vi "Single.vi"() -> ()   [LabVIEW 2017]
doc: "SubVI criada para testar o funcionamento do caso Single Player"
uses:
  controls/DataOut.ctl
  controls/Tabuleiro.ctl
  controls/GameOption.ctl
  controls/States.ctl
  controls/DataIn.ctl
  controls/LogStates.ctl
  controls/TabuleiroCoordenadas.ctl
panel:
  in  "Reiniciar":bool
  in  "Sair":bool
  out "Quem joga":string
  out "Tabuleiro":T1
  out "DataOut":T2
  # "JOGO DA VELHA"
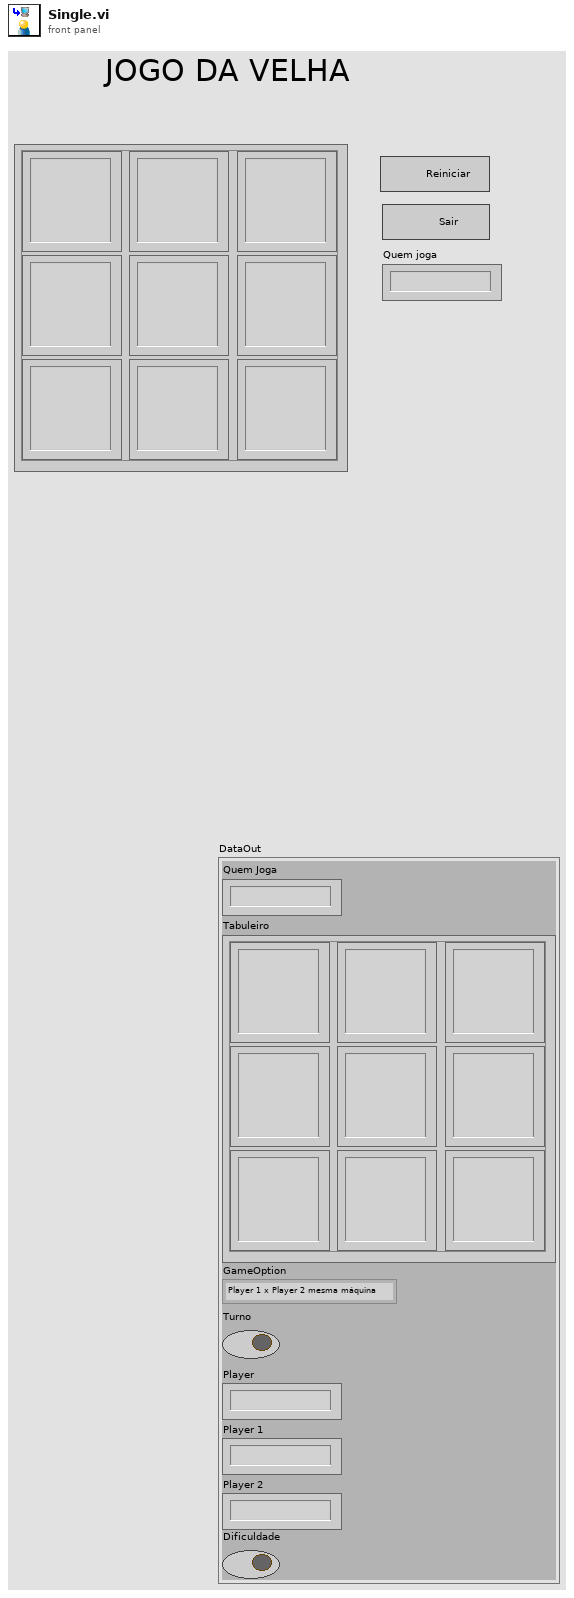
[diagram p1: front panel]
types:
  T1 = typedef "Tabuleiro.ctl" = cluster{"(0,0)":string, "(1,0)":string, "(0,1)":string, "(1,1)":string, "(2,0)":string, "(1,2)":string, "(2,2)":string, "(0,2)":string, "(2,1) ":string}
  T2 = typedef "DataOut.ctl" = cluster{"Quem Joga":string, "Tabuleiro":T1, "GameOption":T3, "Turno":bool, "Player":string, "Player 1":string, "Player 2":string, "Dificuldade":bool}
  T3 = typedef "GameOption.ctl" = enum16{"Player 1 x Player 2 mesma máquina", "Player 1 x Player 2 pela rede", "Player 1 x Computador", "Wait for Event", "Initialize"}
  T4 = typedef "States.ctl" = enum16{"Initialize", "Player (wait for event)", "Stop", "PC", "Restart"}
  T5 = typedef "DataIn.ctl" = cluster{"Quem Joga":string, "Tabuleiro":T1, "GameOption":T3, "Turno":bool, "Player":string, "Player 1":string, "Player 2":string, "Dificuldade":bool}
  T6 = typedef "LogStates.ctl" = enum16{"Initialize", "Write", "Write (win, draw)", "Write (PC first)", "Write (Player first)", "Close"}
  T7 = typedef "TabuleiroCoordenadas.ctl" = enum16{"0,0", "0,1", "0,2", "1,0", "1,1", "1,2", "2,0", "2,1", "2,2"}
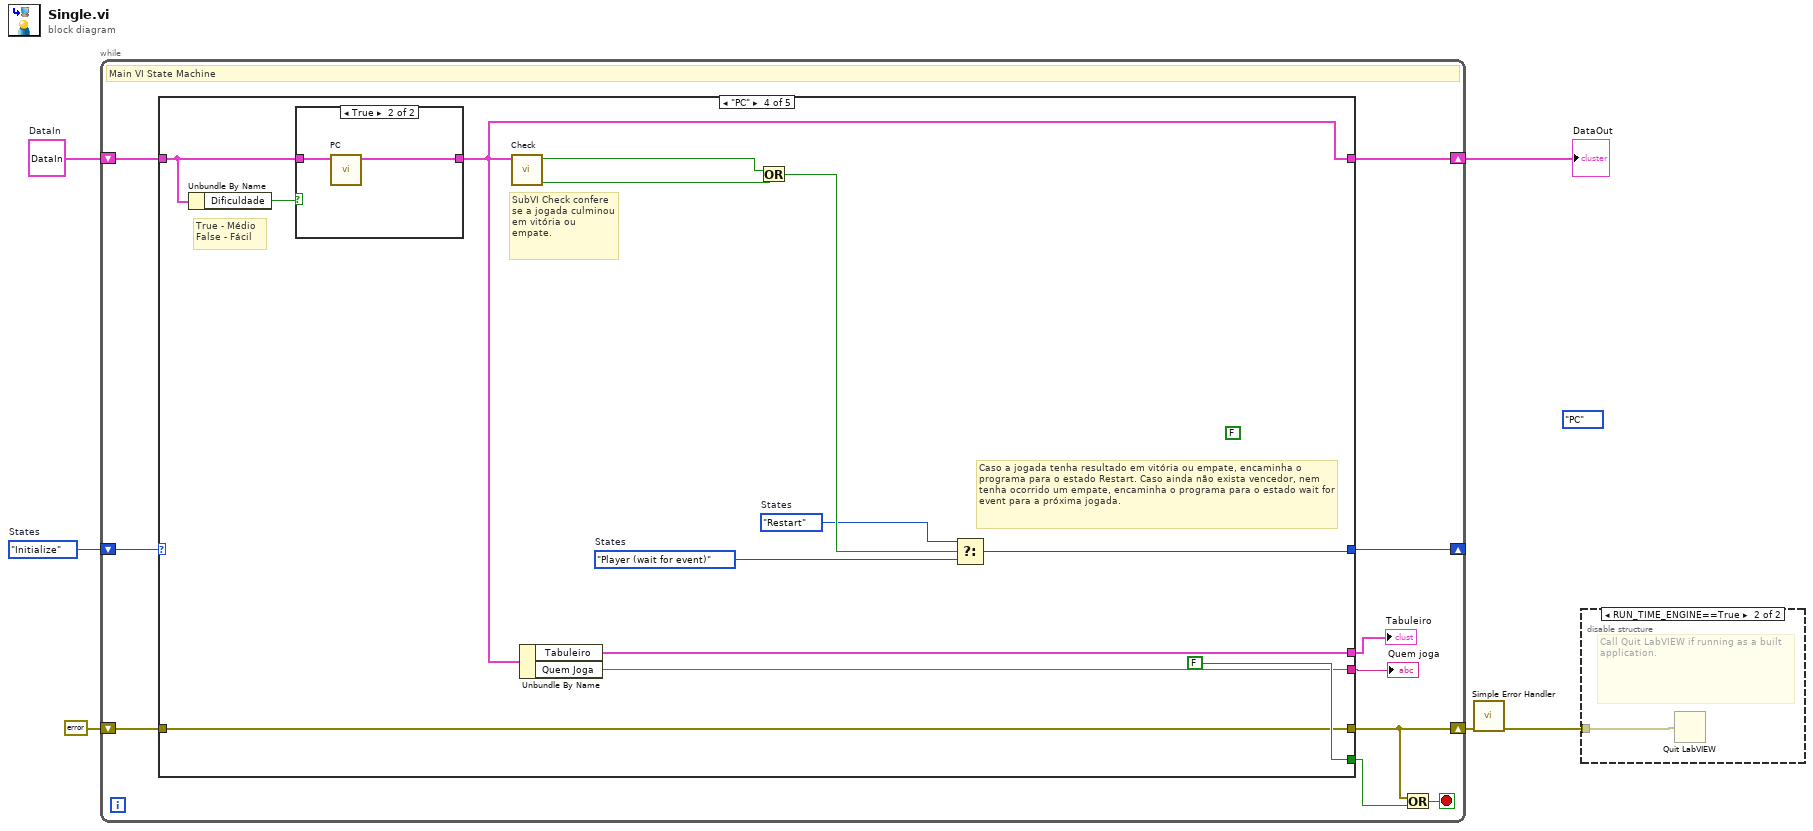
[diagram p0: block diagram]
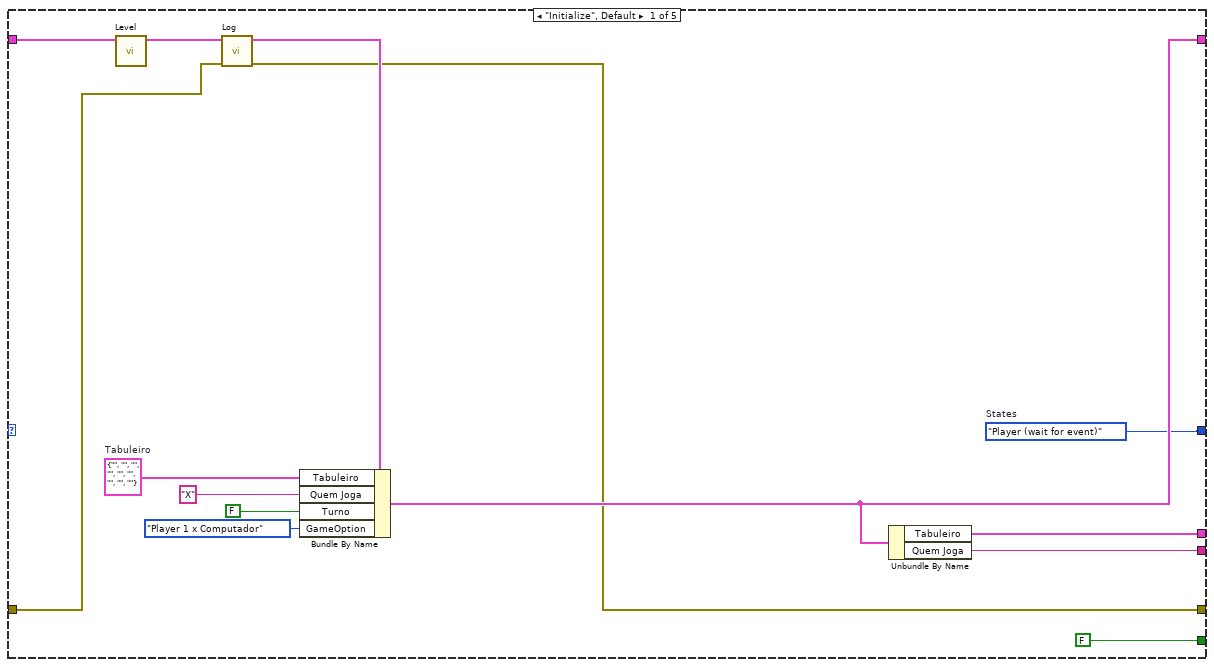
[diagram p3: hidden frame]
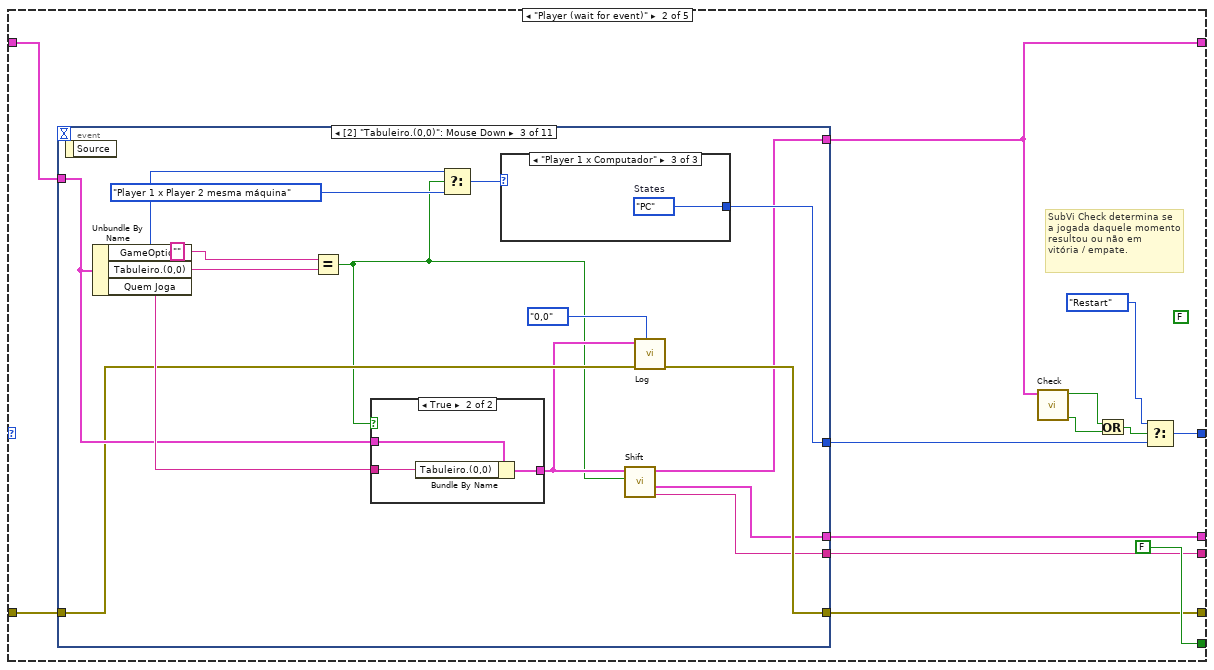
[diagram p4: hidden frame]
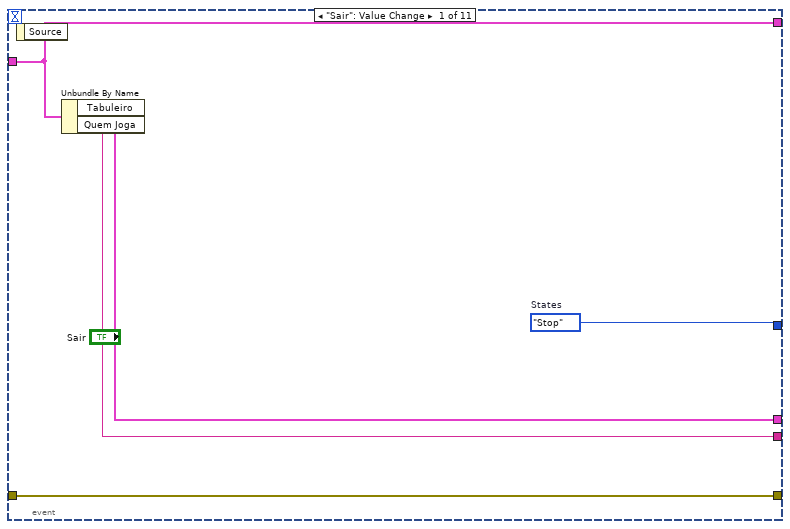
[diagram p5: hidden frame]
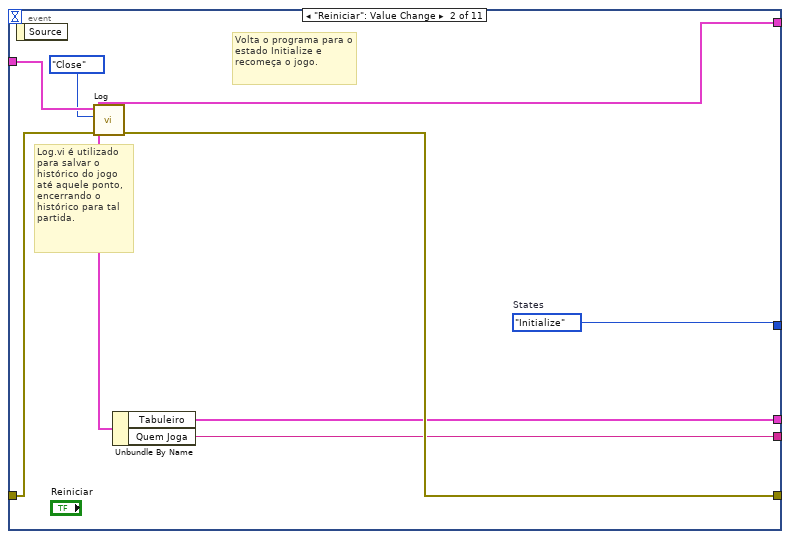
[diagram p6: hidden frame]
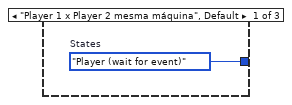
[diagram p8: hidden frame]
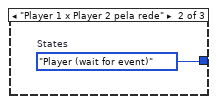
[diagram p9: hidden frame]
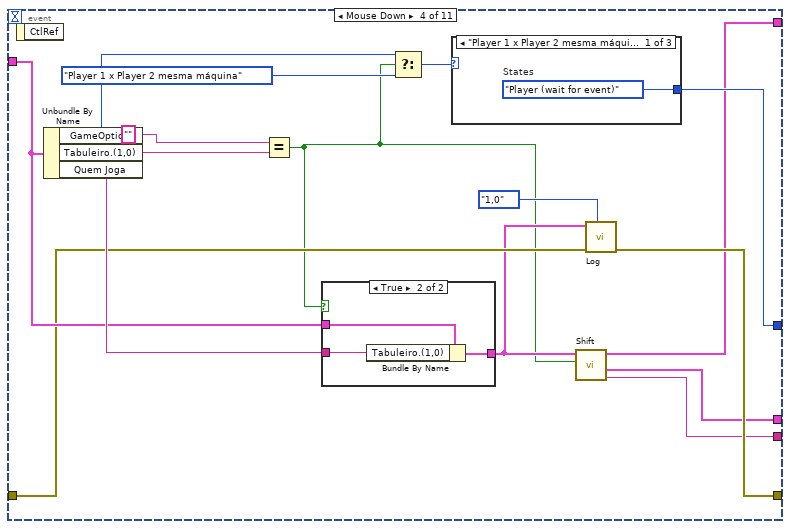
[diagram p10: hidden frame]
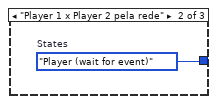
[diagram p12: hidden frame]
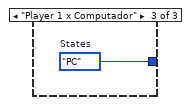
[diagram p13: hidden frame]
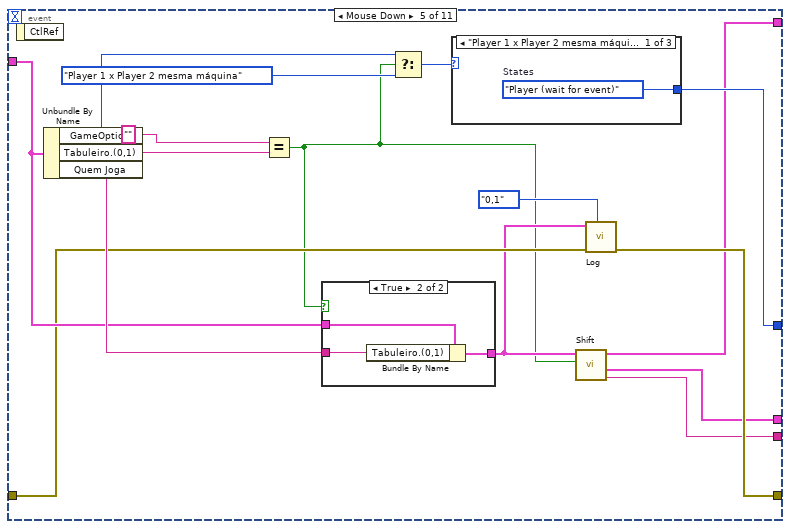
[diagram p14: hidden frame]
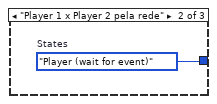
[diagram p16: hidden frame]
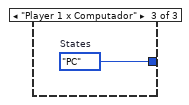
[diagram p17: hidden frame]
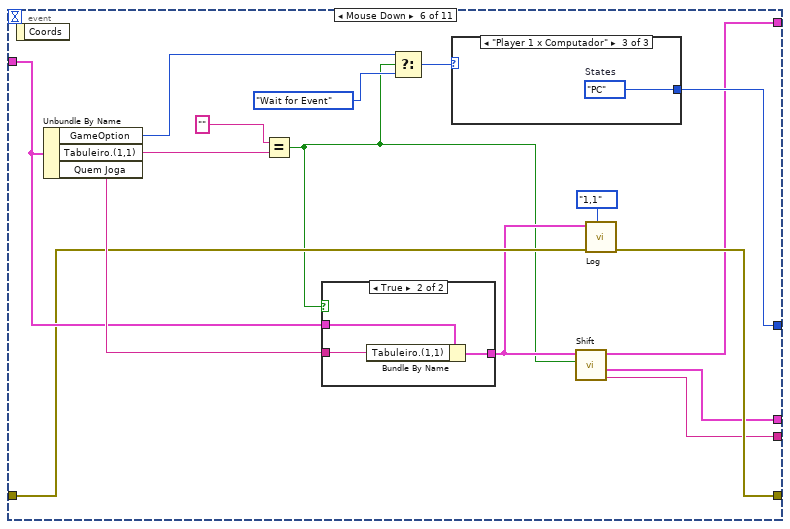
[diagram p18: hidden frame]
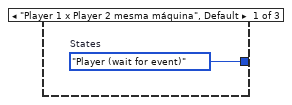
[diagram p20: hidden frame]
diagram:
  (unwired) States."PC" ("f")
  w4 = T5 {"Quem Joga"="", "Tabuleiro"={"(0,0)"="", "(1,0)"="", "(0,1)"="", "(1,1)"="", "(2,0)"="", "(1,2)"="", "(2,2)"="", "(0,2)"="", "(2,1) "=""}, "GameOption"=enum."Player 1 x Player 2 mesma máquina", "Turno"=FALSE, "Player"="", "Player 1"="", "Player 2"="", "Dificuldade"=FALSE}  # DataIn
  w5 = States."Initialize"  # States
  n1 = while {
    shift-right: [w13] -> w6
    shift-left: w4 -> [w14]
    shift-right: [w11] -> w3
    shift-left: errorcluster {"status"=FALSE, "code"=0, "source"=""} ("error constant") -> [w12]
    shift-right: [w10] -> _
    shift-left: w5 -> [w15]
    stop <- w16 stop-if-true
    # "Main VI State Machine"
    n2 = case shown="\"PC\"" w15 {
      tunnel: w14 -> [w18 w42 w267 w271 w296]
      tunnel: [w27 w31 w267 w272 w287] -> w13
      tunnel: w12 -> [w20 w41 w269 w273 w295]
      tunnel: [w19 w40 w269 w273 w288] -> w11
      tunnel: [w23 w36 w268 w276 w289] -> w10
      tunnel: [w26 w39 w266 w275 w293] -> w9
      tunnel: [w25 w38 w265 w274 w292] -> w8
      tunnel: [FALSE FALSE TRUE FALSE FALSE] -> w7
      frame "Initialize", Default {
        w23 = States."Player (wait for event)"  # States
        w28 = T1 {"(0,0)"="", "(1,0)"="", "(0,1)"="", "(1,1)"="", "(2,0)"="", "(1,2)"="", "(2,2)"="", "(0,2)"="", "(2,1) "=""}  # Tabuleiro
        n3 = call "Level.vi"("DataIn"=w18) -> ("Cluster"=w17:T2)  [unwired: 10 in]
        n4 = call "Log.vi"("Error In"=w20, "DataIn"=w17) -> ("Error Out"=w19:errorcluster, "DataOut"=w21:T2)  [unwired: 8 in]
        n5 = Bundle By Name(cluster=w21, "Tabuleiro"=w28, "Quem Joga"="X", "Turno"=FALSE, "GameOption"=GameOption."Player 1 x Computador") -> (w27:T2)
        n6 = Unbundle By Name(w27) -> ("Tabuleiro"=w25:T1, "Quem Joga"=w26:string)
      }
      frame "Player (wait for event)" {
        (unwired) FALSE ("Nível")
        # "SubVi Check determina se a jogada daquele momento resultou ou não em vitória / empate."
        n7 = event shown="[2] \"Tabuleiro.(0,0)\": Mouse Down" {
          selector: _ -> [_ _ _ _ _ _ _ _ _ _ _]
          dyn-events: _ -> [_ _ _ _ _ _ _ _ _ _ _]
          timeout: _ -> [_ _ _ _ _ _ _ _ _ _ _]
          tunnel: w42 -> [w48 w55 w65 w88 w111 w135 w157 w180 w203 w226 w249]
          tunnel: [w48 w51 w60 w83 w106 w130 w152 w175 w198 w221 w244] -> w31
          tunnel: w41 -> [w47 w53 w63 w86 w109 w133 w155 w178 w201 w224 w247]
          tunnel: [w47 w52 w62 w85 w108 w132 w154 w177 w200 w223 w246] -> w40
          tunnel: [w46 w50 w59 w82 w105 w129 w151 w174 w197 w220 w243] -> w38
          tunnel: [w45 w49 w58 w81 w104 w128 w150 w173 w196 w219 w242] -> w39
          tunnel: [w44 w56 w67 w90 w113 w137 w159 w182 w205 w228 w251] -> w37
          event "Sair": Value Change {
            w44 = States."Stop"  # States
            n8 = event-data() -> ()  [unwired: 1 in, 1 out]
            n9 = Unbundle By Name(w48) -> ("Tabuleiro"=w46:T1, "Quem Joga"=w45:string)
          }
          event "Reiniciar": Value Change {
            w56 = States."Initialize"  # States
            # "Log.vi é utilizado para salvar o histórico do jogo até aquele ponto, encerrando o histórico para tal partida."
            # "Volta o programa para o estado Initialize e recomeça o jogo."
            n10 = event-data() -> ()  [unwired: 1 in, 1 out]
            n11 = call "Log.vi"("Error In"=w53, "Log States"=LogStates."Close", "DataIn"=w55) -> ("Error Out"=w52:errorcluster, "DataOut"=w51:T2)  [unwired: 7 in]
            n12 = Unbundle By Name(w51) -> ("Tabuleiro"=w50:T1, "Quem Joga"=w49:string)
          }
          event Mouse Down {
            n13 = event-data() -> ()  [unwired: 1 in, 1 out]
            n14 = Unbundle By Name(w65) -> ("GameOption"=w69:T3, "Tabuleiro.(0,0)"=w72:string, "Quem Joga"=w66:string)
            n15 = Equal?(x="", y=w72) -> (x = y?=w57:bool)
            n16 = case shown="True" w57 {
              tunnel: w66 -> [_ w75]
              tunnel: w65 -> [w73 w76]
              tunnel: [w73 w74] -> w61
              frame False {
              }
              frame True {
                n17 = Bundle By Name(cluster=w76, "Tabuleiro.(0,0)"=w75) -> (w74:T2)
              }
            }
            n18 = Select(t=w69, s=w57, f=GameOption."Player 1 x Player 2 mesma máquina") -> (s? t:f=w68:T3)
            n19 = case shown="\"Player 1 x Computador\"" w68 {
              tunnel: [w77 w78 w79] -> w67
              frame "Player 1 x Player 2 mesma máquina", Default {
                w77 = States."Player (wait for event)"  # States
              }
              frame "Player 1 x Player 2 pela rede" {
                w78 = States."Player (wait for event)"  # States
              }
              frame "Player 1 x Computador" {
                w79 = States."PC"  # States
              }
            }
            n20 = call "Shift.vi"("Confirmação"=w57, "DataIn"=w61) -> ("Turno"=w58:string, "Tabuleiro"=w59:T1, "DataOut"=w60:T2)  [unwired: 7 in]
            n21 = call "Log.vi"("Enum Coordenadas"=TabuleiroCoordenadas."0,0" ("Enum"), "Error In"=w63, "DataIn"=w61) -> ("Error Out"=w62:errorcluster)  [unwired: 7 in, 1 out]
          }
          event Mouse Down {
            n22 = event-data() -> ()  [unwired: 1 in, 1 out]
            n23 = Unbundle By Name(w88) -> ("GameOption"=w92:T3, "Tabuleiro.(1,0)"=w95:string, "Quem Joga"=w89:string)
            n24 = Equal?(x="", y=w95) -> (x = y?=w80:bool)
            n25 = case shown="True" w80 {
              tunnel: w89 -> [_ w98]
              tunnel: w88 -> [w96 w99]
              tunnel: [w96 w97] -> w84
              frame False {
              }
              frame True {
                n26 = Bundle By Name(cluster=w99, "Tabuleiro.(1,0)"=w98) -> (w97:T2)
              }
            }
            n27 = Select(t=w92, s=w80, f=GameOption."Player 1 x Player 2 mesma máquina") -> (s? t:f=w91:T3)
            n28 = case shown="\"Player 1 x Player 2 mesma máquina\", Default" w91 {
              tunnel: [w100 w101 w102] -> w90
              frame "Player 1 x Player 2 mesma máquina", Default {
                w100 = States."Player (wait for event)"  # States
              }
              frame "Player 1 x Player 2 pela rede" {
                w101 = States."Player (wait for event)"  # States
              }
              frame "Player 1 x Computador" {
                w102 = States."PC"  # States
              }
            }
            n29 = call "Shift.vi"("Confirmação"=w80, "DataIn"=w84) -> ("Turno"=w81:string, "Tabuleiro"=w82:T1, "DataOut"=w83:T2)  [unwired: 7 in]
            n30 = call "Log.vi"("Enum Coordenadas"=TabuleiroCoordenadas."1,0" ("Enum"), "Error In"=w86, "DataIn"=w84) -> ("Error Out"=w85:errorcluster)  [unwired: 7 in, 1 out]
          }
          event Mouse Down {
            n31 = event-data() -> ()  [unwired: 1 in, 1 out]
            n32 = Unbundle By Name(w111) -> ("GameOption"=w115:T3, "Tabuleiro.(0,1)"=w118:string, "Quem Joga"=w112:string)
            n33 = Equal?(x="", y=w118) -> (x = y?=w103:bool)
            n34 = case shown="True" w103 {
              tunnel: w112 -> [_ w121]
              tunnel: w111 -> [w119 w122]
              tunnel: [w119 w120] -> w107
              frame False {
              }
              frame True {
                n35 = Bundle By Name(cluster=w122, "Tabuleiro.(0,1)"=w121) -> (w120:T2)
              }
            }
            n36 = Select(t=w115, s=w103, f=GameOption."Player 1 x Player 2 mesma máquina") -> (s? t:f=w114:T3)
            n37 = case shown="\"Player 1 x Player 2 mesma máquina\", Default" w114 {
              tunnel: [w123 w124 w125] -> w113
              frame "Player 1 x Player 2 mesma máquina", Default {
                w123 = States."Player (wait for event)"  # States
              }
              frame "Player 1 x Player 2 pela rede" {
                w124 = States."Player (wait for event)"  # States
              }
              frame "Player 1 x Computador" {
                w125 = States."PC"  # States
              }
            }
            n38 = call "Shift.vi"("Confirmação"=w103, "DataIn"=w107) -> ("Turno"=w104:string, "Tabuleiro"=w105:T1, "DataOut"=w106:T2)  [unwired: 7 in]
            n39 = call "Log.vi"("Enum Coordenadas"=TabuleiroCoordenadas."0,1" ("Enum"), "Error In"=w109, "DataIn"=w107) -> ("Error Out"=w108:errorcluster)  [unwired: 7 in, 1 out]
          }
          event Mouse Down {
            n40 = event-data() -> ()  [unwired: 1 in, 1 out]
            n41 = Unbundle By Name(w135) -> ("GameOption"=w126:T3, "Tabuleiro.(1,1)"=w141:string, "Quem Joga"=w136:string)
            n42 = Equal?(x="", y=w141) -> (x = y?=w127:bool)
            n43 = case shown="True" w127 {
              tunnel: w136 -> [_ w144]
              tunnel: w135 -> [w142 w145]
              tunnel: [w142 w143] -> w131
              frame False {
              }
              frame True {
                n44 = Bundle By Name(cluster=w145, "Tabuleiro.(1,1)"=w144) -> (w143:T2)
              }
            }
            n45 = Select(t=w126, s=w127, f=GameOption."Wait for Event") -> (s? t:f=w138:T3)
            n46 = case shown="\"Player 1 x Computador\"" w138 {
              tunnel: [w146 w147 w148] -> w137
              frame "Player 1 x Player 2 mesma máquina", Default {
                w146 = States."Player (wait for event)"  # States
              }
              frame "Player 1 x Player 2 pela rede" {
                w147 = States."Player (wait for event)"  # States
              }
              frame "Player 1 x Computador" {
                w148 = States."PC"  # States
              }
            }
            n47 = call "Shift.vi"("Confirmação"=w127, "DataIn"=w131) -> ("Turno"=w128:string, "Tabuleiro"=w129:T1, "DataOut"=w130:T2)  [unwired: 7 in]
            n48 = call "Log.vi"("Enum Coordenadas"=TabuleiroCoordenadas."1,1" ("Enum"), "Error In"=w133, "DataIn"=w131) -> ("Error Out"=w132:errorcluster)  [unwired: 7 in, 1 out]
          }
          event Mouse Down {
            n49 = event-data() -> ()  [unwired: 1 in, 1 out]
            n50 = Unbundle By Name(w157) -> ("GameOption"=w161:T3, "Tabuleiro.(2,0)"=w164:string, "Quem Joga"=w158:string)
            n51 = Equal?(x="", y=w164) -> (x = y?=w149:bool)
            n52 = case shown="True" w149 {
              tunnel: w158 -> [_ w167]
              tunnel: w157 -> [w165 w168]
              tunnel: [w165 w166] -> w153
              frame False {
              }
              frame True {
                n53 = Bundle By Name(cluster=w168, "Tabuleiro.(2,0)"=w167) -> (w166:T2)
              }
            }
            n54 = Select(t=w161, s=w149, f=GameOption."Player 1 x Player 2 mesma máquina") -> (s? t:f=w160:T3)
            n55 = case shown="\"Player 1 x Player 2 mesma máquina\", Default" w160 {
              tunnel: [w169 w170 w171] -> w159
              frame "Player 1 x Player 2 mesma máquina", Default {
                w169 = States."Player (wait for event)"  # States
              }
              frame "Player 1 x Player 2 pela rede" {
                w170 = States."Player (wait for event)"  # States
              }
              frame "Player 1 x Computador" {
                w171 = States."PC"  # States
              }
            }
            n56 = call "Shift.vi"("Confirmação"=w149, "DataIn"=w153) -> ("Turno"=w150:string, "Tabuleiro"=w151:T1, "DataOut"=w152:T2)  [unwired: 7 in]
            n57 = call "Log.vi"("Enum Coordenadas"=TabuleiroCoordenadas."2,0" ("Enum"), "Error In"=w155, "DataIn"=w153) -> ("Error Out"=w154:errorcluster)  [unwired: 7 in, 1 out]
          }
          event Mouse Down {
            n58 = event-data() -> ()  [unwired: 1 in, 1 out]
            n59 = Unbundle By Name(w180) -> ("GameOption"=w184:T3, "Tabuleiro.(1,2)"=w187:string, "Quem Joga"=w181:string)
            n60 = Equal?(x="", y=w187) -> (x = y?=w172:bool)
            n61 = case shown="True" w172 {
              tunnel: w181 -> [_ w190]
              tunnel: w180 -> [w188 w191]
              tunnel: [w188 w189] -> w176
              frame False {
              }
              frame True {
                n62 = Bundle By Name(cluster=w191, "Tabuleiro.(1,2)"=w190) -> (w189:T2)
              }
            }
            n63 = Select(t=w184, s=w172, f=GameOption."Player 1 x Player 2 mesma máquina") -> (s? t:f=w183:T3)
            n64 = case shown="\"Player 1 x Player 2 mesma máquina\", Default" w183 {
              tunnel: [w192 w193 w194] -> w182
              frame "Player 1 x Player 2 mesma máquina", Default {
                w192 = States."Player (wait for event)"  # States
              }
              frame "Player 1 x Player 2 pela rede" {
                w193 = States."Player (wait for event)"  # States
              }
              frame "Player 1 x Computador" {
                w194 = States."PC"  # States
              }
            }
            n65 = call "Shift.vi"("Confirmação"=w172, "DataIn"=w176) -> ("Turno"=w173:string, "Tabuleiro"=w174:T1, "DataOut"=w175:T2)  [unwired: 7 in]
            n66 = call "Log.vi"("Enum Coordenadas"=TabuleiroCoordenadas."1,2" ("Enum"), "Error In"=w178, "DataIn"=w176) -> ("Error Out"=w177:errorcluster)  [unwired: 7 in, 1 out]
          }
          event Mouse Down {
            n67 = event-data() -> ()  [unwired: 1 in, 1 out]
            n68 = Unbundle By Name(w203) -> ("GameOption"=w207:T3, "Tabuleiro.(2,2)"=w210:string, "Quem Joga"=w204:string)
            n69 = Equal?(x="", y=w210) -> (x = y?=w195:bool)
            n70 = case shown="True" w195 {
              tunnel: w204 -> [_ w213]
              tunnel: w203 -> [w211 w214]
              tunnel: [w211 w212] -> w199
              frame False {
              }
              frame True {
                n71 = Bundle By Name(cluster=w214, "Tabuleiro.(2,2)"=w213) -> (w212:T2)
              }
            }
            n72 = Select(t=w207, s=w195, f=GameOption."Player 1 x Player 2 mesma máquina") -> (s? t:f=w206:T3)
            n73 = case shown="\"Player 1 x Player 2 mesma máquina\", Default" w206 {
              tunnel: [w215 w216 w217] -> w205
              frame "Player 1 x Player 2 mesma máquina", Default {
                w215 = States."Player (wait for event)"  # States
              }
              frame "Player 1 x Player 2 pela rede" {
                w216 = States."Player (wait for event)"  # States
              }
              frame "Player 1 x Computador" {
                w217 = States."PC"  # States
              }
            }
            n74 = call "Shift.vi"("Confirmação"=w195, "DataIn"=w199) -> ("Turno"=w196:string, "Tabuleiro"=w197:T1, "DataOut"=w198:T2)  [unwired: 7 in]
            n75 = call "Log.vi"("Enum Coordenadas"=TabuleiroCoordenadas."2,2" ("Enum"), "Error In"=w201, "DataIn"=w199) -> ("Error Out"=w200:errorcluster)  [unwired: 7 in, 1 out]
          }
          event Mouse Down {
            n76 = event-data() -> ()  [unwired: 1 in, 1 out]
            n77 = Unbundle By Name(w226) -> ("GameOption"=w230:T3, "Tabuleiro.(0,2)"=w233:string, "Quem Joga"=w227:string)
            n78 = Equal?(x="", y=w233) -> (x = y?=w218:bool)
            n79 = case shown="True" w218 {
              tunnel: w227 -> [_ w236]
              tunnel: w226 -> [w234 w237]
              tunnel: [w234 w235] -> w222
              frame False {
              }
              frame True {
                n80 = Bundle By Name(cluster=w237, "Tabuleiro.(0,2)"=w236) -> (w235:T2)
              }
            }
            n81 = Select(t=w230, s=w218, f=GameOption."Player 1 x Player 2 mesma máquina") -> (s? t:f=w229:T3)
            n82 = case shown="\"Player 1 x Player 2 mesma máquina\", Default" w229 {
              tunnel: [w238 w239 w240] -> w228
              frame "Player 1 x Player 2 mesma máquina", Default {
                w238 = States."Player (wait for event)"  # States
              }
              frame "Player 1 x Player 2 pela rede" {
                w239 = States."Player (wait for event)"  # States
              }
              frame "Player 1 x Computador" {
                w240 = States."PC"  # States
              }
            }
            n83 = call "Shift.vi"("Confirmação"=w218, "DataIn"=w222) -> ("Turno"=w219:string, "Tabuleiro"=w220:T1, "DataOut"=w221:T2)  [unwired: 7 in]
            n84 = call "Log.vi"("Enum Coordenadas"=TabuleiroCoordenadas."0,2" ("Enum"), "Error In"=w224, "DataIn"=w222) -> ("Error Out"=w223:errorcluster)  [unwired: 7 in, 1 out]
          }
          event Mouse Down {
            n85 = event-data() -> ()  [unwired: 1 in, 1 out]
            n86 = Unbundle By Name(w249) -> ("GameOption"=w253:T3, "Tabuleiro.(2,1)"=w256:string, "Quem Joga"=w250:string)
            n87 = Equal?(x="", y=w256) -> (x = y?=w241:bool)
            n88 = case shown="True" w241 {
              tunnel: w250 -> [_ w259]
              tunnel: w249 -> [w257 w260]
              tunnel: [w257 w258] -> w245
              frame False {
              }
              frame True {
                n89 = Bundle By Name(cluster=w260, "Tabuleiro.(2,1)"=w259) -> (w258:T2)
              }
            }
            n90 = Select(t=w253, s=w241, f=GameOption."Player 1 x Player 2 mesma máquina") -> (s? t:f=w252:T3)
            n91 = case shown="\"Player 1 x Player 2 mesma máquina\", Default" w252 {
              tunnel: [w261 w262 w263] -> w251
              frame "Player 1 x Player 2 mesma máquina", Default {
                w261 = States."Player (wait for event)"  # States
              }
              frame "Player 1 x Player 2 pela rede" {
                w262 = States."Player (wait for event)"  # States
              }
              frame "Player 1 x Computador" {
                w263 = States."PC"  # States
              }
            }
            n92 = call "Shift.vi"("Confirmação"=w241, "DataIn"=w245) -> ("Turno"=w242:string, "Tabuleiro"=w243:T1, "DataOut"=w244:T2)  [unwired: 7 in]
            n93 = call "Log.vi"("Enum Coordenadas"=TabuleiroCoordenadas."2,1" ("Enum"), "Error In"=w247, "DataIn"=w245) -> ("Error Out"=w246:errorcluster)  [unwired: 7 in, 1 out]
          }
        }
        n94 = call "Check.vi"("DataIn"=w31) -> ("True = Empatou"=w34:bool, "True = Ganhou"=w33:bool)  [unwired: 9 in]
        n95 = Or(x=w33, y=w34) -> (x .or. y?=w32:bool)
        n96 = Select(t=States."Restart", s=w32, f=w37) -> (s? t:f=w36:T4)
      }
      frame "Stop" {
        w268 = States."Stop"  # States
        n97 = Unbundle By Name(w267) -> ("Tabuleiro"=w265:T1, "Quem Joga"=w266:string)
      }
      frame "PC" {
        (unwired) FALSE ("Nível")
        w277 = States."Player (wait for event)"  # States
        w278 = States."Restart"  # States
        # "True - Médio\nFalse - Fácil"
        # "Caso a jogada tenha resultado em vitória ou empate, encaminha o programa para o estado Restart. Caso ainda não exista vencedor, nem tenha ocorrido um empate, encaminha o programa para o estado wait for event para a próxima jogada."
        # "SubVI Check confere se a jogada culminou em vitória ou empate."
        n98 = Unbundle By Name(w271) -> ("Dificuldade"=w270:bool)
        n99 = case shown="True" w270 {
          tunnel: w271 -> [w283 w286]
          tunnel: [w284 w285] -> w272
          frame False {
            n100 = call "SimpleMove.vi"("DataIn"=w283) -> ("DataOut"=w284:T2)  [unwired: 10 in]
          }
          frame True {
            n101 = call "PC.vi"("DataIn"=w286) -> ("DataOut"=w285:T2)  [unwired: 10 in]
          }
        }
        n102 = call "Check.vi"("DataIn"=w272) -> ("True = Empatou"=w280:bool, "True = Ganhou"=w281:bool)  [unwired: 9 in]
        n103 = Unbundle By Name(w272) -> ("Tabuleiro"=w274:T1, "Quem Joga"=w275:string)
        n104 = Or(x=w281, y=w280) -> (x .or. y?=w279:bool)
        n105 = Select(t=w278, s=w279, f=w277) -> (s? t:f=w276:T4)
      }
      frame "Restart" {
        (unwired) FALSE ("Nível")
        n106 = call "Check.vi"("DataIn"=w296) -> ("True = Empatou"=w297:bool)  [unwired: 9 in, 1 out]
        n107 = case shown="True" w297 {
          tunnel: w296 -> [w301 w315]
          tunnel: w295 -> [w300 w314]
          tunnel: [w300 w314] -> w294
          tunnel: [w304 w313] -> w292
          tunnel: [w303 w312] -> w293
          tunnel: [w299 w311] -> w291
          tunnel: [States."Initialize" ("States") w310] -> w289
          frame False {
            n108 = Unbundle By Name(w301) -> ("Tabuleiro"=w304:T1, "Quem Joga"=w303:string, "Turno"=w305:bool)
            n109 = case shown="False" w305 {
              tunnel: w301 -> [w307 w309]
              tunnel: [w306 w308] -> w299
              frame False {
                n110 = call "O.vi"("DataIn"=w307) -> ("DataOut"=w306:T2)  [unwired: 10 in]
              }
              frame True {
                n111 = call "X.vi"("DataIn"=w309) -> ("DataOut"=w308:T2)  [unwired: 10 in]
              }
            }
          }
          frame True {
            w310 = States."Initialize"  # States
            n112 = call "Draw.vi"("DataIn"=w315) -> ("DataOut"=w311:T2)  [unwired: 10 in]
            n113 = Unbundle By Name(w311) -> ("Tabuleiro"=w313:T1, "Quem Joga"=w312:string)
          }
        }
        n114 = call "Log.vi"("Error In"=w294, "Log States"=LogStates."Write (win, draw)", "DataIn"=w291) -> ("Error Out"=w288:errorcluster, "DataOut"=w287:T2)  [unwired: 7 in]
      }
    }
    "Quem joga" <- w9
    "Tabuleiro" <- w8
    n115 = Or(x=w11, y=w7) -> (x .or. y?=w16:bool)
  }
  "DataOut" <- w6
  n116 = call <vilib>:"Simple Error Handler.vi"("error in (no error)"=w3) -> ("error out"=w1:errorcluster)  [unwired: 4 in, 4 out]
  n117 = disable-structure shown="RUN_TIME_ENGINE==True" {
    disable-tunnel: w1 -> [_ w316]
    frame condition #0 (active) {
    }
    frame condition #1 {
      # "Call Quit LabVIEW if running as a built application."
      n118 = Quit LabVIEW(quit? (T)=w316) -> ()
    }
  }
